vi "Brower Unit Test.vi"   [LabVIEW 2015, in "Browers Controller.lvclass"]
uses:
  Brower Controller/Browers Controller.lvclass
  <vilib>/ActorFramework/Actor/Actor.lvclass
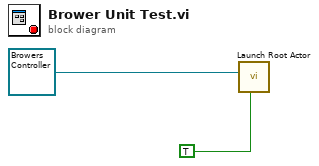
[diagram p0: block diagram]
diagram:
  n1 = call <vilib>:"Launch Root Actor.vi"("Open Actor Core front panel? (F)"=TRUE, "Actor"=refnum<class "Browers Controller.lvclass"> refnum ("Browers")) -> ()  [unwired: 8 in, 2 out]
